vi "Performance Init and Generation Test.vi"() -> ()   [LabVIEW 2021]
doc: "Measure the average duration of <b>Init Erro Handler</b> with 1000 error codes XML at the input and average <b>Generate Error</b> duration with no input to format."
panel:
  out "Avg Generation Duration [ms]":dbl
  out "Avg Init Duration [ms]":dbl
  in  "error in":errorcluster
  # "Measure the average duration of Init Erro Handler with 1000 error codes XML at the input and average Generate Error duration with no input to format."
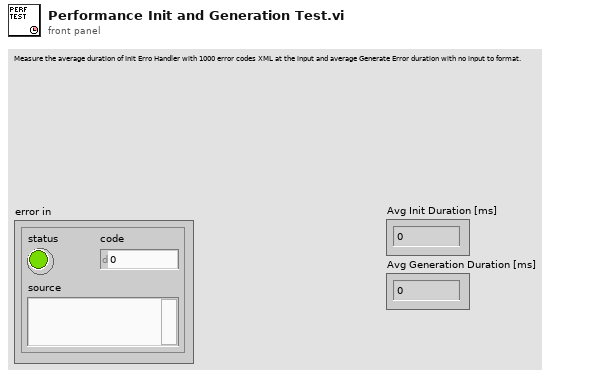
[diagram p1: front panel]
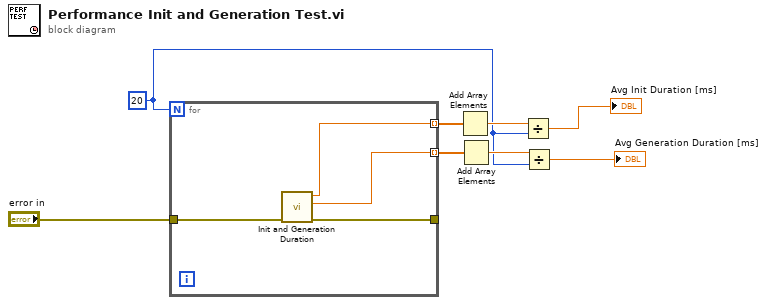
[diagram p0: block diagram]
diagram:
  w4 = 20
  n1 = for {
    N: w4 -> [_]
    tunnel: [w12] -> _
    tunnel: "error in" -> [w11]
    tunnel: [w10] -> w8 mode=indexing
    tunnel: [w9] -> w7 mode=indexing
    n2 = call "Init and Generation Duration.vi"("error in"=w11) -> ("Generated Error"=w12:errorcluster, "Generation Duration [ms]"=w9:dbl, "Init Duration [ms]"=w10:dbl)  [unwired: 8 in]
  }
  n3 = Add Array Elements(numeric array=w8) -> (sum=w6:dbl)
  n4 = Add Array Elements(numeric array=w7) -> (sum=w5:dbl)
  n5 = Divide(x=w6, y=w4) -> (x/y=→"Avg Init Duration [ms]":dbl)
  n6 = Divide(x=w5, y=w4) -> (x/y=→"Avg Generation Duration [ms]":dbl)
